vi "Analysis.LevelTransition.OPH.vi"(9 "Array in":dbl[][](array[numeric]), 10 "LVTransitionParameters":T1, 11 "Numeric":dbl) -> (2 "Results":dbl[](array[numeric]), 3 "Array out":bool[](array[boolean]))   [LabVIEW 2015, in "TestStand Analysis Steps.lvlib"]
uses:
  TestStand Analysis Steps.lvlib
  Types/Public.LVAnalysis.ctl
  Types/Public.ChLVAnalysis.ctl
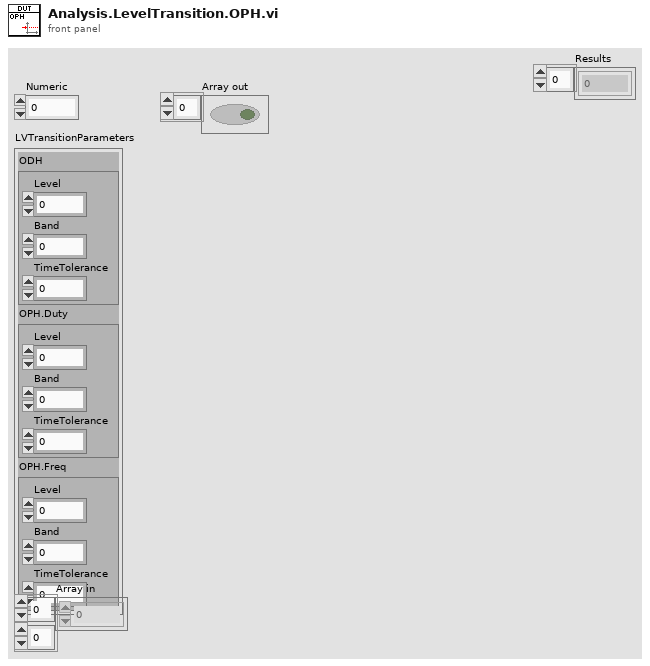
[diagram p1: front panel]
types:
  T1 = typedef "TestStand Analysis Steps.lvlib/Public.LVAnalysis.ctl" = cluster{"ODH":T2, "OPH.Duty":T2, "OPH.Freq":T2}
  T2 = typedef "TestStand Analysis Steps.lvlib/Public.ChLVAnalysis.ctl" = cluster{"Level":dbl, "Band":dbl, "TimeTolerance":dbl}
  T3 = cluster{"Scale":dbl, "Hi":dbl, "Lo":dbl, "dt":dbl, "Timeout":dbl}
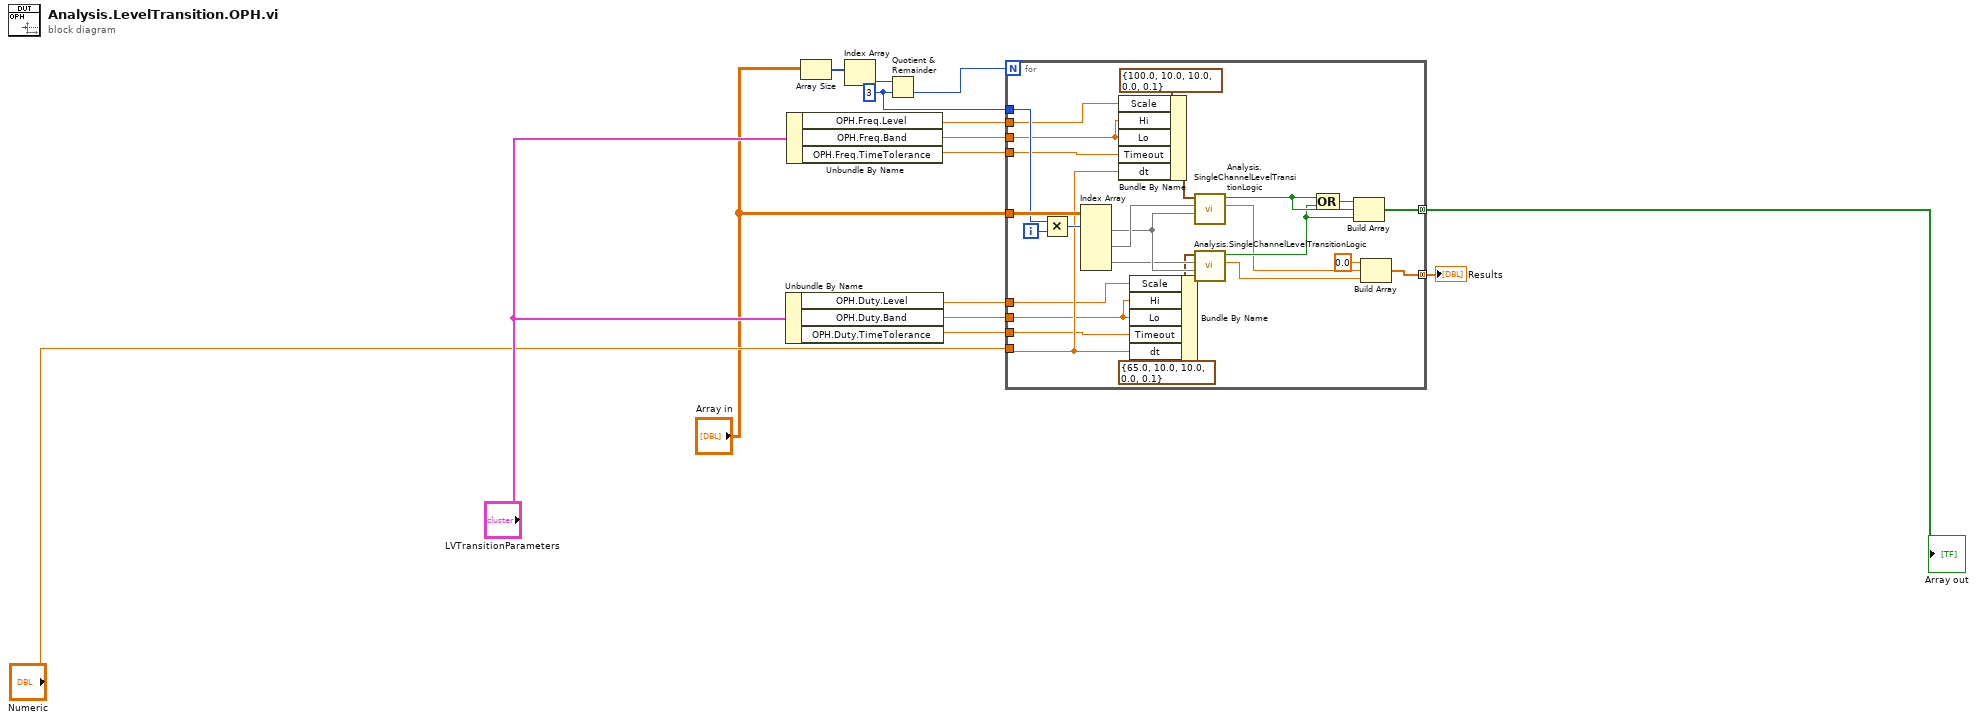
[diagram p0: block diagram]
diagram:
  w2 = 3 ("y")
  n1 = Unbundle By Name("LVTransitionParameters") -> ("OPH.Duty.Level"=w14:dbl, "OPH.Duty.Band"=w13:dbl, "OPH.Duty.TimeTolerance"=w12:dbl)
  n2 = Unbundle By Name("LVTransitionParameters") -> ("OPH.Freq.Level"=w11:dbl, "OPH.Freq.Band"=w10:dbl, "OPH.Freq.TimeTolerance"=w9:dbl)
  n3 = Array Size(array="Array in") -> (size(s)=w5:i32[])
  n4 = Index Array(array=w5) -> (element=w4:i32)  [unwired: 1 in]
  n5 = Quotient & Remainder(x=w4, y=w2) -> (floor(x/y)=w3:i32)  [unwired: 1 out]
  n6 = for {
    N: w3 -> [_]
    tunnel: "Array in" -> [w41]
    tunnel: w2 -> [w36]
    tunnel: [w35] -> w7 mode=concatenating
    tunnel: "Numeric" -> [w26]
    tunnel: w9 -> [w25]
    tunnel: w10 -> [w24]
    tunnel: w11 -> [w23]
    tunnel: w12 -> [w22]
    tunnel: w13 -> [w21]
    tunnel: w14 -> [w20]
    tunnel: [w17] -> w1 mode=concatenating
    i -> [w38]
    n7 = Multiply(x=w36, y=w38) -> (x*y=w37:i32)
    n8 = Index Array(array=w41, index (row) #1=w37) -> (element #1=w34:dbl[], element #2=w39:dbl[], element #3=w33:dbl[])  [unwired: 5 in]
    n9 = Bundle By Name(cluster=T3 {"Scale"=100.0, "Hi"=10.0, "Lo"=10.0, "dt"=0.0, "Timeout"=0.1} ("Parameters"), "Scale"=w23, "Hi"=w24, "Lo"=w24, "Timeout"=w25, "dt"=w26) -> (w40:T3)
    n10 = Bundle By Name(cluster=T3 {"Scale"=65.0, "Hi"=10.0, "Lo"=10.0, "dt"=0.0, "Timeout"=0.1} ("Parameters"), "Scale"=w20, "Hi"=w21, "Lo"=w21, "Timeout"=w22, "dt"=w26) -> (w31:T3)
    n11 = call "Analysis.SingleChannelLevelTransitionLogic.vi"("Stimulus"=w34, "Response"=w39, "Parameters"=w40) -> ("Result"=w19:dbl, "Fail"=w29:bool)  [unwired: 7 in]
    n12 = call "Analysis.SingleChannelLevelTransitionLogic.vi"("Stimulus"=w34, "Response"=w33, "Parameters"=w31) -> ("Result"=w18:dbl, "Fail"=w28:bool)  [unwired: 7 in]
    n13 = Compound Arithmetic op=OR(w29, w28) -> (w27:bool)
    n14 = Build Array(w27, w29, w28) -> (w35:bool[])
    n15 = Build Array(0.0 ("element"), w19, w18) -> (w17:dbl[])
  }
  "Array out" <- w7
  "Results" <- w1
